vi "Create New Source Distribution.vi"(7 "TargetItem Refnum":refnum<vi>, 8 "error in (no error)":errorcluster, 10 "Build specification name":string, 11 "Project Refnum":refnum<vi>) -> (0 "error out":errorcluster, 3 "SDIST out":refnum<class "NI_AB_API_SDIST.lvclass">)   [LabVIEW 2020, in "NI_AB_API_SDIST.lvclass"]
uses:
  <vilib>/AppBuilder/AB_API/SDIST/NI_AB_API_SDIST.lvclass
  e:/builds/penguin/labview/branches/2020/dev/dist/vi.lib/AppBuilder/AB_API/Build/NI_AB_API_Build.lvclass
  <vilib>/AppBuilder/AB_API/common/AB_API Compiled Code Option.ctl
  <vilib>/AppBuilder/AB_Classes/SourceDistribution/AB_SourceDistribution.lvclass
  e:/builds/penguin/labview/branches/2020/dev/dist/vi.lib/AppBuilder/AB_Classes/Build/AB_Build.lvclass
  <vilib>/AppBuilder/AB_API/common/AB_API Build Object Type.ctl
  <vilib>/AppBuilder/AB_API/Build/NI_AB_API_Build.lvclass
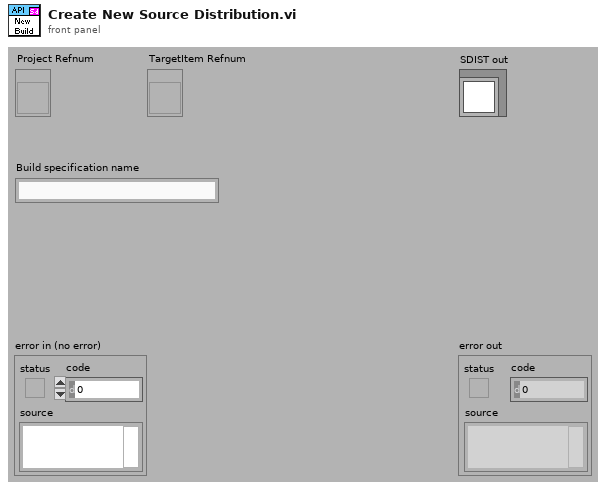
[diagram p1: front panel]
types:
  T1 = typedef "AB_API Compiled Code Option.ctl" = enum16{"Preserve compiled code", "Remove compiled code", "Preserve file settings"}
  T2 = typedef "AB_API Build Object Type.ctl" = enum16{"Source Distribution", "DLL", "EXE", "Installer", "Zip File", "RESTful WS", "RTEXE", "Packed Library", "C Generation ", ".NET Interop Assembly"}
  T3 = typedef "ItemRef.ctl" = u64
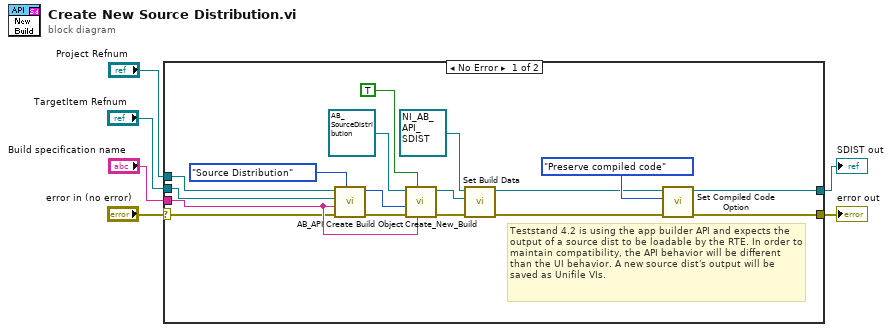
[diagram p0: block diagram]
diagram:
  n1 = case shown="No Error" "error in (no error)" {
    selector: "error in (no error)" -> [w21 w24]
    tunnel: [w7 w24] -> w5
    tunnel: [w9 _] -> w4
    tunnel: "Build specification name" -> [w23 _]
    tunnel: "TargetItem Refnum" -> [w22 _]
    tunnel: "Project Refnum" -> [w19 _]
    frame No Error {
      # "Teststand 4.2 is using the app builder API and expects the output of a source dist to be loadable by the RTE. In order to maintain compatibility, the API behavior will be different than the UI behavior. A new source dist's output will be saved as Unifile VIs."
      n2 = call <vilib>:"AB_API Create Build Object.vi"("Build object type"=AB_API_Build_Object_Type."Source Distribution", "error in (no error)"=w21, "Build spec name"=w23, "TargetItem Refnum"=w22, "Project Refnum"=w19) -> ("error out"=w17:errorcluster, "Build object"=w18:T3)  [unwired: 5 in]
      n3 = call-dynamic "Create_New_Build.vi"("buildSpecName"=w23, "Programmatic? (false)"=TRUE, "error in (no error)"=w17, "buildObject"=w18, "AB_SourceDistribution in"=refnum<class "AB_SourceDistribution.lvclass"> refnum) -> ("error out"=w12:errorcluster, "AB_SourceDistribution out"=w13:refnum<class "AB_SourceDistribution.lvclass">)  [unwired: 5 in]
      n4 = call <vilib>:"Set Build Data.vi"("error in (no error)"=w12, "AB_Build.lvclass"=w13, "NI_AB_API_Build in"=refnum<class "NI_AB_API_SDIST.lvclass"> refnum ("AB_API_SDIST.lvclass")) -> ("error out"=w8:errorcluster, "NI_AB_API_Build out"=w10:refnum<class "NI_AB_API_SDIST.lvclass">)  [unwired: 7 in]
      n5 = call-dynamic "Set Compiled Code Option.vi"("error in (no error)"=w8, "Compiled code option"=AB_API_Compiled_Code_Option."Preserve compiled code", "NI_AB_API_SDIST in"=w10) -> ("error out"=w7:errorcluster, "NI_AB_API_SDIST out"=w9:refnum<class "NI_AB_API_SDIST.lvclass">)  [unwired: 7 in]
    }
    frame Error {
    }
  }
  "error out" <- w5
  "SDIST out" <- w4
